vi "Read XML.vi"(8 "error in":errorcluster, 11 "selected path":path) -> (0 "error out":errorcluster caption="error in", 3 "Custom Device reference out":refnum<k24>)   [LabVIEW 2015, in "Configuration Tool.lvlib"]
uses:
  NationalInstruments.VeriStand.XMLReader
  <vilib>/Utility/sysdir.llb/System Directory Type.ctl
  subVI/Config Global.vi
  <vilib>/regexp/Match Regular Expression.xnode
  Configuration Tool.lvlib
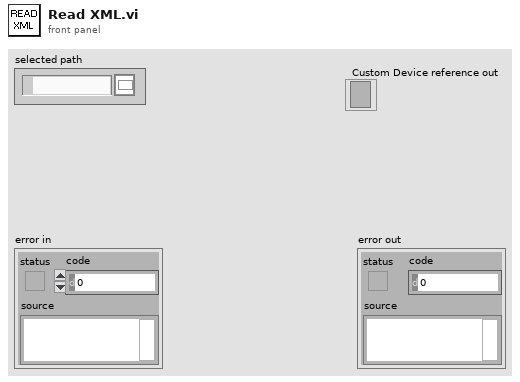
[diagram p1: front panel]
types:
  T1 = typedef "System Directory Type.ctl" = i32
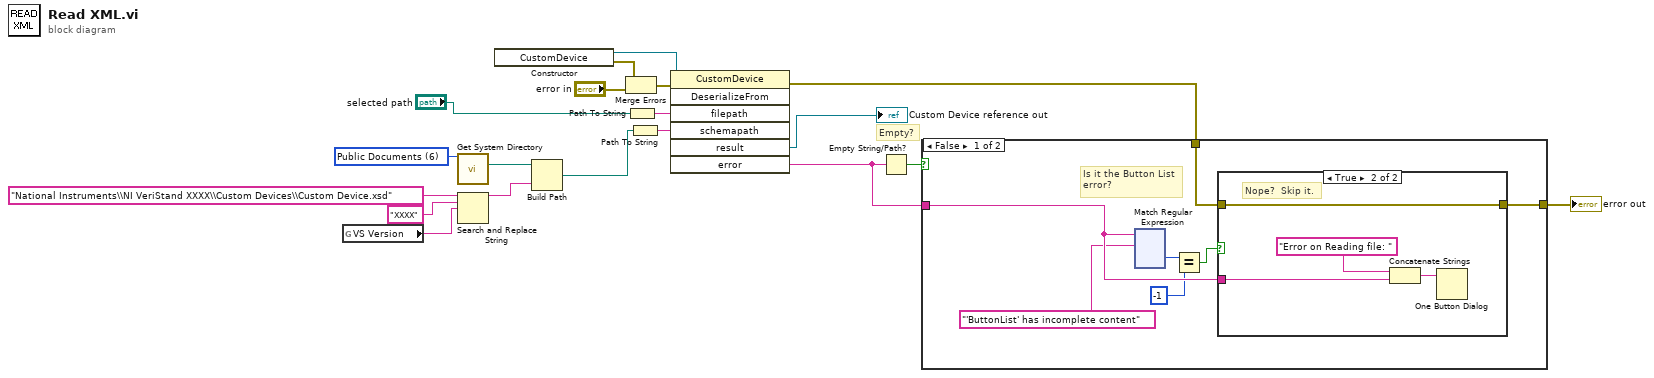
[diagram p0: block diagram]
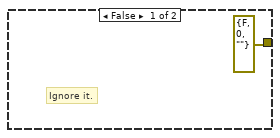
[diagram p2: hidden frame]
diagram:
  w13 = T1 6 items=["User Home"=0, "User Desktop"=1, "User Documents"=2, "User Application Data"=3, "User Preferences"=4, "User Temporary"=5, "Public Documents"=6, "Public Application Data"=7, "Public Preferences"=8, "Public Cache"=13, "System Core Libraries"=9, "System Installed Libraries"=10, "Application Files"=11, "Boot Volume Root"=12] ("system directory type")
  # "Empty?"
  n1 = global read "Config Global.vi" "VS Version"() -> (w2:string)
  n2 = call <vilib>:"Get System Directory.vi"("system directory type"=w13) -> ("system directory"=w12:path)  [unwired: 10 in]
  n3 = Search and Replace String(input string="National Instruments\\NI VeriStand XXXX\\Custom Devices\\Custom Device.xsd", search string="XXXX", replace string=w2) -> (result string=w1:string)  [unwired: 5 in, 3 out]
  n4 = constructor class="CustomDevice"() -> (reference out=w15:refnum<k24>, error out=w9:errorcluster)  [unwired: 3 in, 1 out]
  n5 = Build Path(base path=w12, name or relative path=w1) -> (appended path=w11:path)
  n6 = Merge Errors(w9, "error in") -> (w8:errorcluster)
  n7 = Path To String(path="selected path") -> (string=w14:string)
  n8 = Path To String(path=w11) -> (string=w10:string)
  n9 = invoke class="CustomDevice" method="DeserializeFrom"(reference=w15, error in=w8, "filepath"=w14, "schemapath"=w10) -> (error out=w5:errorcluster, "result"=→"Custom Device reference out":refnum<k24>, "error"=w7:string)  [unwired: 3 in, 4 out]
  n10 = Empty String/Path?(string/path=w7) -> (empty?=w6:bool)
  n11 = case shown="False" w6 {
    tunnel: w7 -> [w26 _]
    tunnel: w5 -> [w22 w143]
    tunnel: [w21 w143] -> w18
    frame False {
      # "Is it the Button List\nerror?"
      n12 = xnode "Match Regular Expression"("input string"=w26, "regular expression"="'ButtonList' has incomplete content") -> ("offset past match"=w24:i32)  [unwired: 4 in, 4 out]
      n13 = Equal?(x=w24, y=-1) -> (x = y?=w20:bool)
      n14 = case shown="True" w20 {
        tunnel: w26 -> [_ w29]
        tunnel: w22 -> [_ w28]
        tunnel: [errorcluster {"status"=FALSE, "code"=0, "source"=""} ("error out") w28] -> w21
        frame False {
          # "Ignore it."
        }
        frame True {
          # "Nope?  Skip it."
          n15 = Concatenate Strings("Error on Reading file: " ("string"), w29) -> (w31:string)
          n16 = One Button Dialog(message=w31) -> ()  [unwired: 1 in, 1 out]
        }
      }
    }
    frame True {
    }
  }
  "error out" <- w18
